vi "EnqueueDrive.vi"(8 "error in (no error)":errorcluster, 10 "LoopTiming":u32, 11 "DriveInstruction":T1) -> (0 "error out":errorcluster)   [LabVIEW 2013]
uses:
  DriveInstruction.ctl
  DriveQueueInstruction.ctl
  QueueSubsystem.ctl
  TankDriveAction.ctl
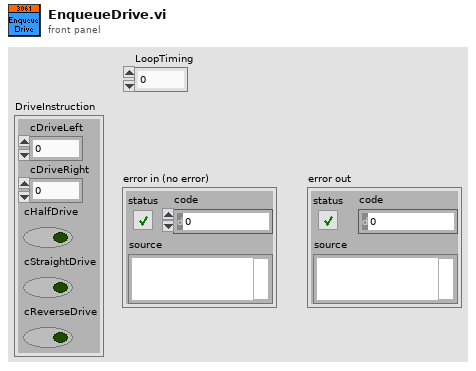
[diagram p1: front panel]
types:
  T1 = typedef "DriveInstruction.ctl" = cluster{"cDriveLeft":dbl, "cDriveRight":dbl, "cHalfDrive":bool, "cStraightDrive":bool, "cReverseDrive":bool}
  T2 = typedef "TankDriveAction.ctl" = enum16{"Init", "LinearDrive", "SetValue", "Disable"}
  T3 = typedef "QueueSubsystem.ctl" = enum16{"Drive", "Arm", "Catapult", "Roller"}
  T4 = typedef "DriveQueueInstruction.ctl" = cluster{"DriveInstruction":T1, "Subsystem":T3, "Action":T2, "LoopTiming":u32}
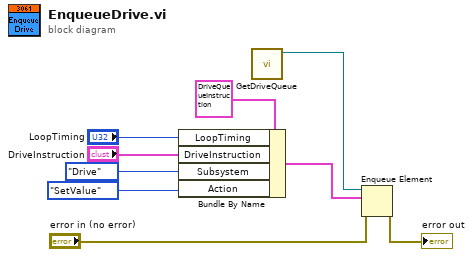
[diagram p0: block diagram]
diagram:
  n1 = Bundle By Name(cluster=T4 {"DriveInstruction"={"cDriveLeft"=0.0, "cDriveRight"=1.0, "cHalfDrive"=FALSE, "cStraightDrive"=FALSE, "cReverseDrive"=FALSE}, "Subsystem"=enum."Arm", "Action"=enum."Init", "LoopTiming"=0} ("DriveQueueInstruction"), "LoopTiming"="LoopTiming", "DriveInstruction"="DriveInstruction", "Subsystem"=QueueSubsystem."Drive", "Action"=TankDriveAction."SetValue") -> (w4:T4)
  n2 = call "GetDriveQueue.vi"() -> ("queue out"=w7:refnum<queue>)  [unwired: 10 in, 1 out]
  n3 = Enqueue Element(queue=w7, element=w4, error in (no error)="error in (no error)") -> (error out=→"error out":errorcluster)  [unwired: 1 in, 2 out]
